vi "Status.Builder.Get State.vi"(11 "Status.Builder in":refnum<class "Status.Builder.lvclass">) -> (2 "Builder State":refnum<class "Status.Builder.State.lvclass">, 3 "Status.Builder out":refnum<class "Status.Builder.lvclass">)   [LabVIEW 2016, in "DSF.Engine.lvlib" / "Status.Builder.lvclass"]
uses:
  Status.Builder.lvclass
  Status.Builder.State.lvclass
  Status.Builder.lvclass/Status.Builder.ctl
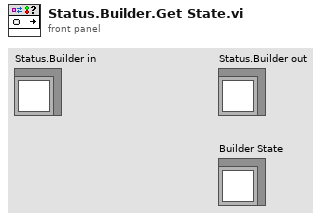
[diagram p1: front panel]
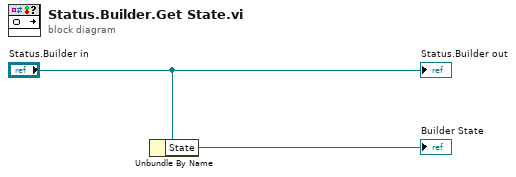
[diagram p0: block diagram]
diagram:
  n1 = Unbundle By Name("Status.Builder in") -> ("State"=→"Builder State":refnum<class "Status.Builder.State.lvclass">)
  "Status.Builder out" <- "Status.Builder in"
